vi "cleanSpool.vi"(8 "error in (no error)":errorcluster, 10 "Total Img Num":i32, 11 "strPath":string="_groundtruth_") -> (0 "error out":errorcluster)   [LabVIEW 2018]
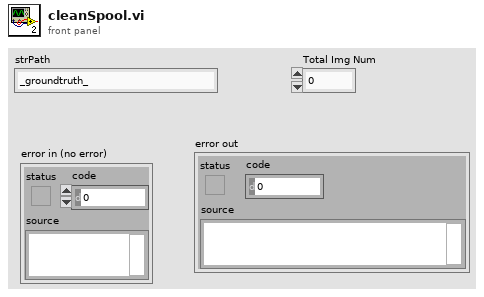
[diagram p1: front panel]
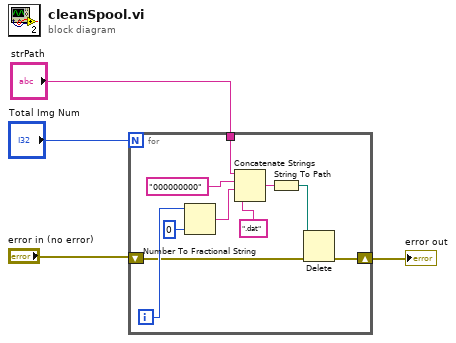
[diagram p0: block diagram]
diagram:
  n1 = for {
    N: "Total Img Num" -> [_]
    tunnel: "strPath" -> [w7]
    shift-right: [w5] -> w2
    shift-left: "error in (no error)" -> [w6]
    i -> [w12]
    n2 = Number To Fractional String(number=w12, precision (6)=0) -> (F-format string=w10:string)  [unwired: 2 in]
    n3 = Concatenate Strings(w7, "000000000", w10, ".dat") -> (w9:string)
    n4 = String To Path(string=w9) -> (path=w14:path)
    n5 = Delete(path (use dialog)=w14, error in=w6) -> (error out=w5:errorcluster)  [unwired: 3 in, 2 out]
  }
  "error out" <- w2
